vi "TcpServer Init.vi"(8 "error in (no error)":errorcluster, 9 "local port":u16, 10 "Driver to run":refnum<class "BaseDriver.lvclass">, 11 "TcpServer in":refnum<class "TcpServer.lvclass">) -> (0 "error out":errorcluster, 3 "TcpServer out":refnum<class "TcpServer.lvclass">)   [LabVIEW 2013, in "TcpServer.lvclass"]
doc: "Initializes the TCP server with a local port to listen to and a driver object that will be cloned and executed for each incoming connection."
uses:
  TcpServer.lvclass
  Driver/BaseDriver/BaseDriver.lvclass
  TcpServer.lvclass/TcpServer.ctl
  Interface/TCP/TCP/TCP.lvclass
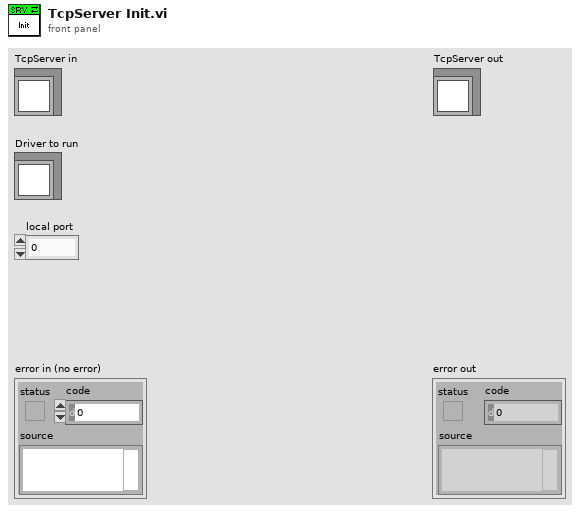
[diagram p1: front panel]
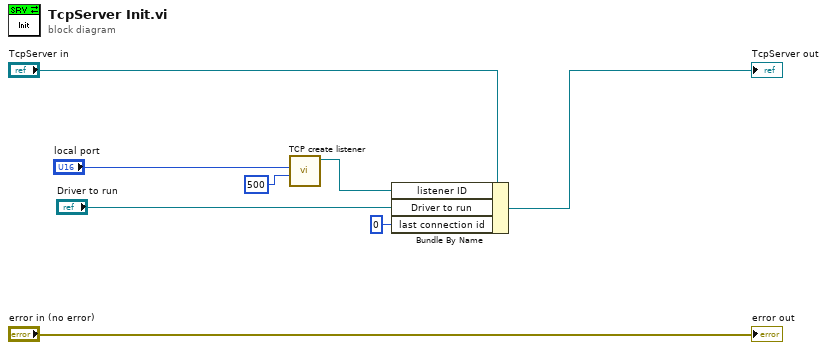
[diagram p0: block diagram]
diagram:
  n1 = call "TCP create listener.vi"("timeout ms (25000)"=500, "port"="local port") -> ("TCP out"=w1:refnum<class "TCP.lvclass">)  [unwired: 7 in, 2 out]
  n2 = Bundle By Name(cluster="TcpServer in", "listener ID"=w1, "Driver to run"="Driver to run", "last connection id"=0) -> (→"TcpServer out":refnum<class "TcpServer.lvclass">)
  "error out" <- "error in (no error)"
